vi "隐藏.vi"(0 "Tab Control":refnum<vi>, 2 "visible":bool=TRUE) -> ()   [LabVIEW 2015]
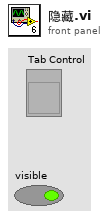
[diagram p1: front panel]
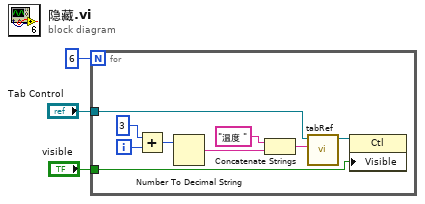
[diagram p0: block diagram]
diagram:
  n1 = for {
    N: 6 -> [_]
    tunnel: "Tab Control" -> [w11]
    tunnel: "visible" -> [w4]
    i -> [w9]
    n2 = Add(x=3, y=w9) -> (x+y=w8:i32)
    n3 = Number To Decimal String(number=w8) -> (decimal integer string=w6:string)  [unwired: 1 in]
    n4 = Concatenate Strings("温度 ", w6) -> (w5:string)
    n5 = call "tabRef.vi"("control name"=w5, "Tab Control"=w11) -> ("control refnum"=w12:refnum<vi>)  [unwired: 8 in, 1 out]
    n6 = property class="Ctl"(reference=w12, "Visible"=w4) -> ()  [unwired: 1 in, 2 out]
  }
